vi "Generate_Training_Data.vi"() -> ()   [LabVIEW 2024]
uses:
  <vilib>/Utility/file.llb/Write Delimited Spreadsheet (DBL).vi
panel:
  in  "File Path":path
  in  "Start Hour":dbl
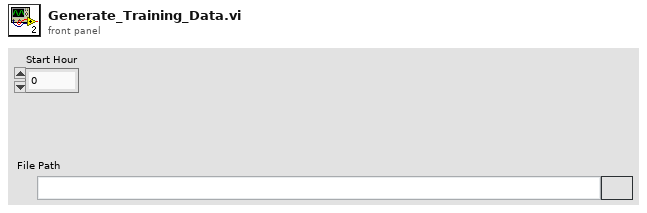
[diagram p1: front panel]
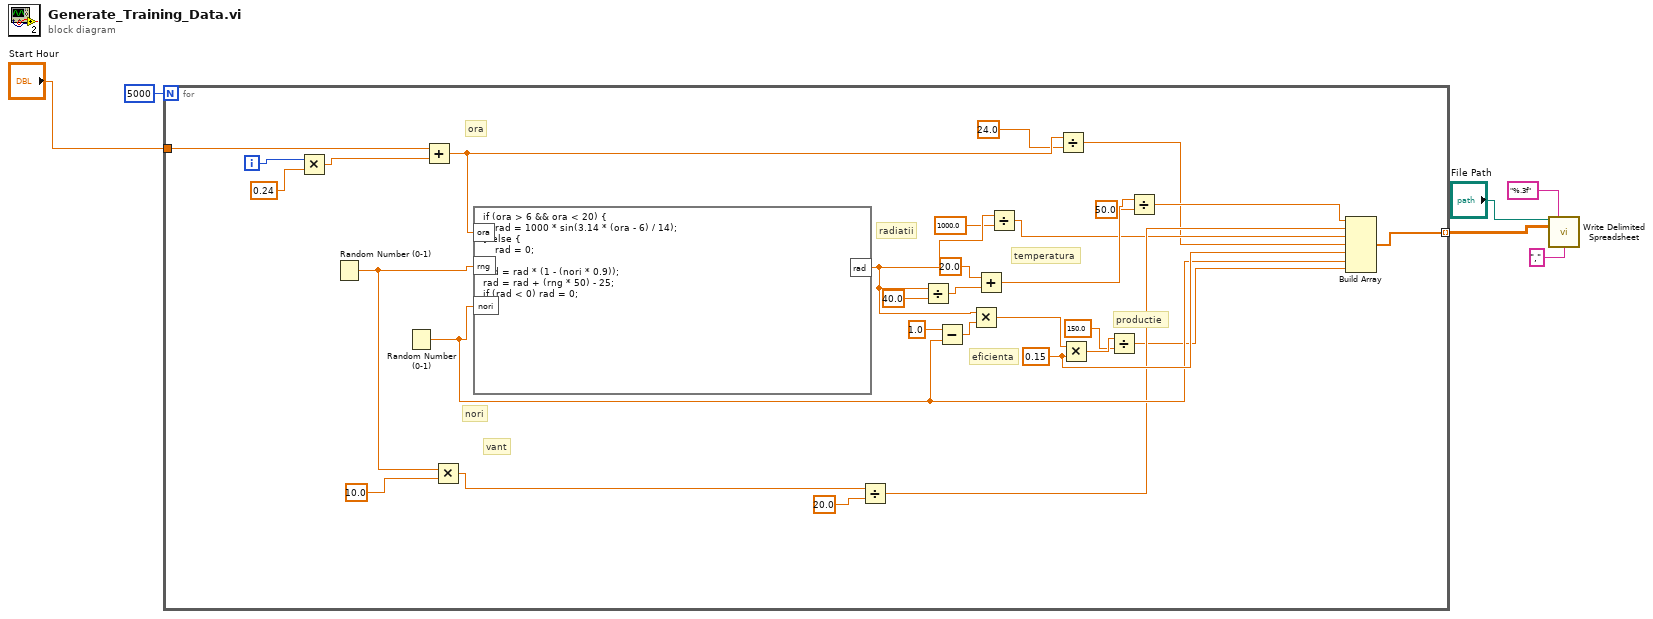
[diagram p0: block diagram]
diagram:
  n1 = for {
    N: 5000 -> [_]
    tunnel: "Start Hour" -> [w33]
    tunnel: [w27] -> w5 mode=indexing
    i -> [w36]
    w26 = 0.15 ("y")
    # "productie"
    # "nori"
    # "temperatura"
    # "eficienta"
    # "ora"
    # "vant"
    # "radiatii"
    n2 = Multiply(x=w36, y=0.24) -> (x*y=w34:dbl)
    n3 = Random Number (0-1)() -> (number: 0 to 1=w29:dbl)
    n4 = Random Number (0-1)() -> (number: 0 to 1=w24:dbl)
    n5 = Add(x=w33, y=w34) -> (x+y=w11:dbl)
    n6 = Multiply(x=w29, y=10.0) -> (x*y=w18:dbl)
    n7 = formula code="if (ora > 6 && ora < 20) {\n    rad = 1000 * sin(3.14 * (ora - 6) / 14);\n} else {\n    rad = 0;\n}\nrad = rad * (1 - (nori * 0.9));\nrad = rad + (rng * 50) - 25;\nif (rad < 0) rad = 0;"("ora"=w11, "rng"=w29, "nori"=w24) -> ("rad"=w15:dbl)
    n8 = Divide(x=w18, y=20.0) -> (x/y=w16:dbl)
    n9 = Divide(x=w15, y=40.0) -> (x/y=w31:dbl)
    n10 = Subtract(x=1.0, y=w24) -> (x-y=w23:dbl)
    n11 = Multiply(x=w15, y=w23) -> (x*y=w22:dbl)
    n12 = Add(x=20.0, y=w31) -> (x+y=w21:dbl)
    n13 = Divide(x=w15, y=1000.0) -> (x/y=w13:dbl)
    n14 = Divide(x=w11, y=24.0) -> (x/y=w12:dbl)
    n15 = Multiply(x=w22, y=w26) -> (x*y=w8:dbl)
    n16 = Divide(x=w8, y=150.0) -> (x/y=w9:dbl)
    n17 = Divide(x=w21, y=50.0) -> (x/y=w19:dbl)
    n18 = Build Array(w19, w16, w13, w12, w26, w24, w9) -> (w27:dbl[])
  }
  n19 = call-poly <vilib>:"Write Delimited Spreadsheet.vi"("file path (dialog if empty)"="File Path", "format (%.3f)"="%.3f", "2D data"=w5, "delimiter (\\t)"="," ("delimiter (\\t)")) -> ()  [unwired: 10 in, 2 out]
